vi "Login Rmb User.vi"(8 "error in (no error)":errorcluster, 10 "rmb user":bool, 11 "INF of [V] Login in":refnum<class "INF of [V] Login.lvclass">) -> (0 "error out":errorcluster, 3 "INF of [V] Login out":refnum<class "INF of [V] Login.lvclass">)   [LabVIEW 2020, in "[V] Login.lvlib" / "INF of [V] Login.lvclass"]
uses:
  INF of [V] Login.lvclass
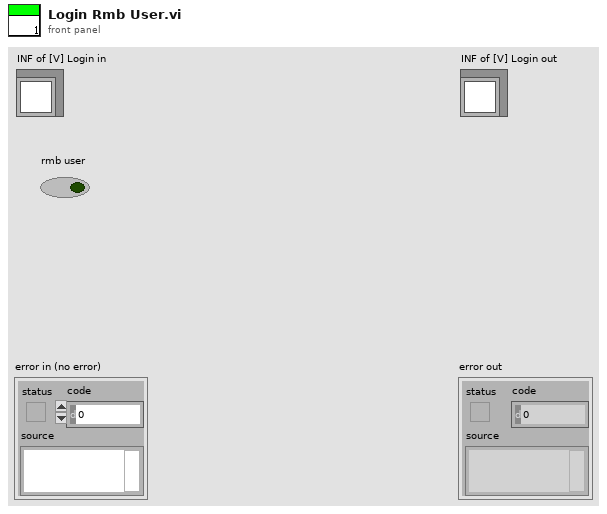
[diagram p1: front panel]
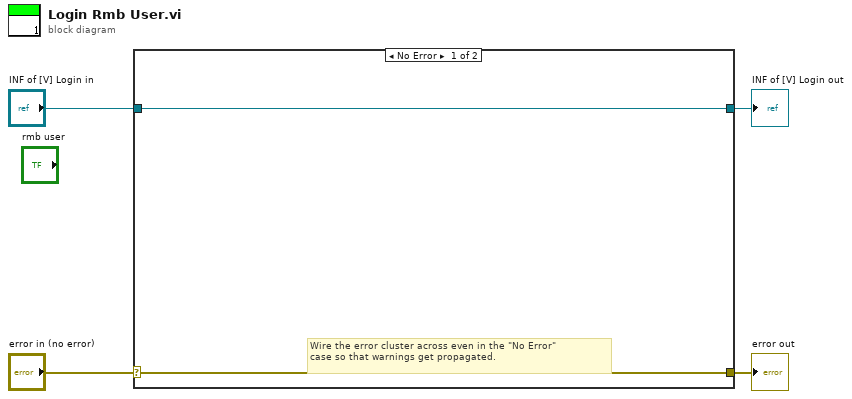
[diagram p0: block diagram]
diagram:
  n1 = case shown="No Error" "error in (no error)" {
    selector: "error in (no error)" -> [w5 w8]
    tunnel: [w5 w8] -> w3
    tunnel: [w6 w7] -> w1
    tunnel: "INF of [V] Login in" -> [w6 w7]
    frame No Error {
      # "Wire the error cluster across even in the \"No Error\"\ncase so that warnings get propagated."
    }
    frame Error {
    }
  }
  "error out" <- w3
  "INF of [V] Login out" <- w1
